vi "연속 읽기 응답 Parsing.vi"(1 "응답 프레임":string="\u000600RSB016430313233323330303233303032333030323330303233303000000000000000000000000000000000000000000000000000000000000000000000000000000000000000000000000000000000000000000000000000000000000000000000000000000000\u0003") -> (0 "배열":u32[](array[numeric]) format="%.0x")   [LabVIEW 2014]
panel:
  out "데이터 개수(문자열)":string
  out "데이터 개수(숫자형)":u32
  out "부분 문자열":string
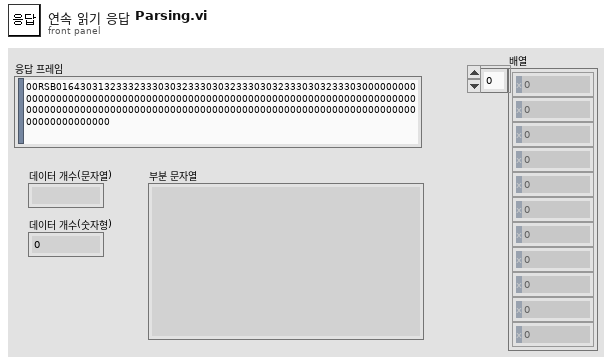
[diagram p1: front panel]
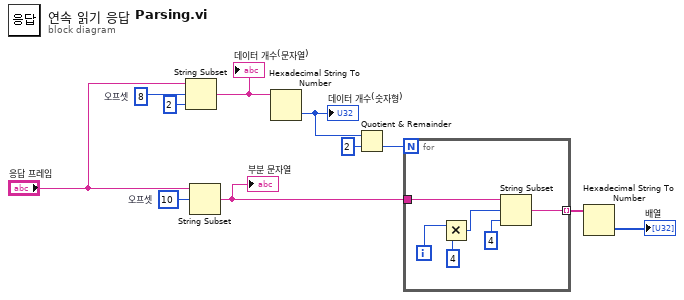
[diagram p0: block diagram]
diagram:
  w9 = 8  # 오프셋
  w11 = 10  # 오프셋
  n1 = String Subset(string="응답 프레임", offset (0)=w9, length (rest)=2 ("길이(나머지)")) -> (substring=w7:string)
  "데이터 개수(문자열)" <- w7
  n2 = String Subset(string="응답 프레임", offset (0)=w11) -> (substring=w3:string)  [unwired: 1 in]
  "부분 문자열" <- w3
  n3 = Hexadecimal String To Number(string=w7) -> (number=w6:u32)  [unwired: 2 in, 1 out]
  "데이터 개수(숫자형)" <- w6
  n4 = Quotient & Remainder(x=w6, y=u32 2) -> (floor(x/y)=w4:u32)  [unwired: 1 out]
  n5 = for {
    N: w4 -> [_]
    tunnel: w3 -> [w13]
    tunnel: [w12] -> w2 mode=indexing
    i -> [w17]
    n6 = Multiply(x=w17, y=4) -> (x*y=w15:i32)
    n7 = String Subset(string=w13, offset (0)=w15, length (rest)=4 ("y")) -> (substring=w12:string)
  }
  n8 = Hexadecimal String To Number(string=w2) -> (number=→"배열":u32[])  [unwired: 2 in, 1 out]
